vi "mod_Modulo Integrator.vi"   [LabVIEW 2020, in "niAMT.lvlib"]
uses:
  <vilib>/addons/Modulation/niAMT.lvlib
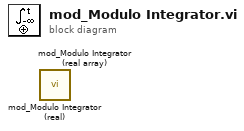
[diagram p0: block diagram]
diagram:
  n1 = call <vilib>:"mod_Modulo Integrator (real).vi"() -> ()  [unwired: 11 in, 1 out]
  n2 = call <vilib>:"mod_Modulo Integrator (real array).vi"() -> ()  [unwired: 11 in, 1 out]
